vi "G4SubTemplate_Simple_6x8x6_NoneModifing.vi"(0 "reference in":refnum<class "G4SubTemplate_Simple_6x8x6.lvclass">, 5 "Error In":errorcluster) -> (14 "reference out":refnum<class "G4SubTemplate_Simple_6x8x6.lvclass">, 19 "Error Out":errorcluster)   [LabVIEW 2020]
uses:
  <resource>/Framework/Providers/Open_GDS/ClassProviders/Provider_EndevoGOOP400/Templates/G4SubTemplate_Simple_6x8x6/G4SubTemplate_Simple_6x8x6.lvclass
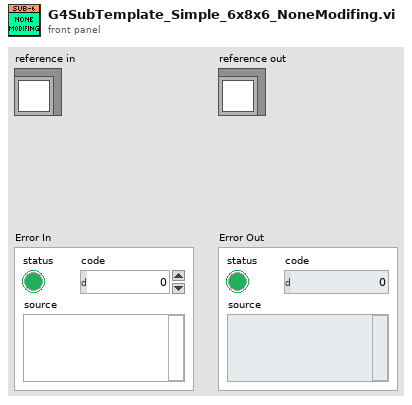
[diagram p1: front panel]
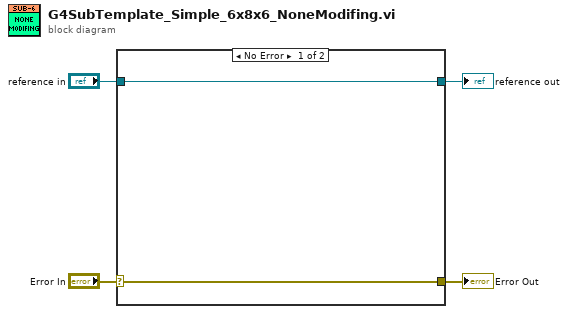
[diagram p0: block diagram]
diagram:
  n1 = case shown="No Error" "Error In" {
    selector: "Error In" -> [w5 w8]
    tunnel: [w5 w8] -> w3
    tunnel: [w6 w7] -> w1
    tunnel: "reference in" -> [w6 w7]
    frame No Error {
    }
    frame Error {
    }
  }
  "Error Out" <- w3
  "reference out" <- w1
